vi "4_Analog_Meter_Reader(Evaluation).vi"() -> ()   [LabVIEW 2020]
uses:
  Controls/Regression_Report.ctl
  <vilib>/Ngene/DeepLTK/Toolkit/NN_Network/Controls/NN_Save_Before_Destroy_Options.ctl
  <vilib>/Ngene/DeepLTK/Toolkit/NN_Network/subVIs/NN_Predict/NN_Predict(In3D_Out1D).vi
  <vilib>/Ngene/DeepLTK/Toolkit/NN_Train/Eval_Loss/NN_Eval_Test_Error_Loss/NN_Eval(In3D_Out1D).vi
  <vilib>/Ngene/DeepLTK/Toolkit/Deep_Learning_Toolkit_by_Ngene.lvlib
panel:
  in  "Image Folder(Test)":path=path "D:/DeepLTK_Examples/Analog_Meter/Test/Images"
  in  "Labels (Test)":path=path "D:/DeepLTK_Examples/Analog_Meter/Test/Labels.csv"
  in  "NN Device":enum16{"CPU", "GPU"}(ring)=enum."GPU"
  in  "Image Folder(Train)":path=path "D:/DeepLTK_Examples/Analog_Meter/Train/Images"
  in  "Labels (Train)":path=path "D:/DeepLTK_Examples/Analog_Meter/Train/Labels.csv"
  out "Metrics (Test)":T1={"Graphs"=[{"Best Linear Fit"=[0.0, 0.7035179734230042, 1.407034993171692, 2.110553026199341, 2.814069986343384, 3.517587900161743, 4.221106052398682, 4.924623012542725, 5.628140926361084, 6.331657886505127, 7.035175800323486, 7.7386932373046875, 8.442211151123047, 9.145729064941406, 9.84924602508545, 10.552763938903809, 11.256280899047852, 11.959798812866211, 12.66331672668457, 13.366833686828613, 14.070351600646973, 14.773868560791016, 15.477387428283691, 16.180904388427734, 16.884422302246094, 17.587940216064453, 18.29145622253418, 18.99497413635254, 19.6984920501709, 20.402009963989258, 21.105527877807617, 21.809045791625977, 22.512563705444336, 23.216079711914062, 23.919597625732422, 24.62311553955078, 25.32663345336914, 26.0301513671875, 26.733667373657227, 27.437185287475586, 28.140703201293945, 28.844221115112305, 29.547739028930664, 30.251256942749023, 30.954774856567383, 31.65829086303711, 32.36180877685547, 33.06532669067383, 33.76884460449219, 34.47236251831055, 35.175880432128906, 35.879398345947266, 36.582916259765625, 37.28643035888672, 37.98994827270508, 38.69346618652344, 39.3969841003418, 40.100502014160156, 40.804019927978516, 41.507537841796875, 42.211055755615234, 42.914573669433594, 43.61809158325195, 44.32160949707031, 45.02512741088867, 45.728641510009766, 46.432159423828125, 47.135677337646484, 47.839195251464844, 48.5427131652832, 49.24623107910156, 49.94974899291992, 50.65326690673828, 51.35678482055664, 52.060302734375, 52.76382064819336, 53.46733856201172, 54.17085266113281, 54.87437057495117, 55.57788848876953, 56.28140640258789, 56.98492431640625, 57.68844223022461, 58.39196014404297, 59.09547805786133, 59.79899597167969, 60.50251388549805, 61.206031799316406, 61.909549713134766, 62.61306381225586, 63.31658172607422, 64.02010345458984, 64.72361755371094, 65.42713928222656, 66.13065338134766, 66.83416748046875, 67.53768920898438, 68.24120330810547, 68.9447250366211, 69.64823913574219, 70.35176086425781, 71.0552749633789, 71.75879669189453, 72.46231079101562, 73.16583251953125, 73.86934661865234, 74.57286071777344, 75.27638244628906, 75.97989654541016, 76.68341827392578, 77.38693237304688, 78.0904541015625, 78.7939682006836, 79.49748992919922, 80.20100402832031, 80.90452575683594, 81.60803985595703, 82.31156158447266, 83.01507568359375, 83.71858978271484, 84.42211151123047, 85.12562561035156, 85.82914733886719, 86.53266143798828, 87.2361831665039, 87.939697265625, 88.64321899414062, 89.34673309326172, 90.05024719238281, 90.75376892089844, 91.45728302001953, 92.16080474853516, 92.86431884765625, 93.56784057617188, 94.27135467529297, 94.9748764038086, 95.67839050292969, 96.38191223144531, 97.0854263305664, 97.78894805908203, 98.49246215820312, 99.19597625732422, 99.89949798583984, 100.60301208496094, 101.30653381347656, 102.01004791259766, 102.71356964111328, 103.41708374023438, 104.12060546875, 104.8241195678711, 105.52764129638672, 106.23115539550781, 106.9346694946289, 107.63819122314453, 108.34170532226562, 109.04522705078125, 109.74874114990234, 110.45226287841797, 111.15577697753906, 111.85929870605469, 112.56281280517578, 113.2663345336914, 113.9698486328125, 114.67337036132812, 115.37688446044922, 116.08039855957031, 116.78392028808594, 117.48743438720703, 118.19095611572266, 118.89447021484375, 119.59799194335938, 120.30150604248047, 121.0050277709961, 121.70854187011719, 122.41206359863281, 123.1155776977539, 123.819091796875, 124.52261352539062, 125.22612762451172, 125.92964935302734, 126.63316345214844, 127.33668518066406, 128.0402069091797, 128.74371337890625, 129.44723510742188, 130.1507568359375, 130.85427856445312, 131.5577850341797, 132.2613067626953, 132.96482849121094, 133.6683349609375, 134.37185668945312, 135.07537841796875, 135.77890014648438, 136.48240661621094, 137.18592834472656, 137.8894500732422, 138.5929718017578, 139.29647827148438, 140.0], "Array 3"=[3.275964, 3.249447, 2.547323, 2.4843557, 2.314022, 5.9284067, 5.9090176, 6.770803, 7.256697, 8.836181, 9.031486, 10.445968, 11.187589, 9.598534, 10.856343, 11.660367, 12.432229, 13.276137, 15.303519, 15.652077, 15.5077095, 15.784932, 16.294615, 17.2778, 18.094921, 18.929054, 19.75645, 20.359539, 20.938688, 22.076456, 22.729862, 23.16336, 23.454283, 24.118996, 25.31959, 26.342335, 26.424267, 26.912985, 27.571787, 28.408794, 29.294344, 30.003319, 30.542835, 31.343233, 32.022118, 32.687912, 33.300972, 34.221542, 34.977905, 35.367214, 36.47949, 37.113617, 37.63445, 37.84932, 38.15908, 40.29969, 40.538902, 40.899334, 41.505558, 42.122498, 42.90602, 43.561836, 44.778614, 44.878468, 45.97382, 46.838966, 47.30163, 47.776108, 48.446632, 48.980473, 49.125286, 50.393486, 51.820633, 52.201366, 52.935173, 53.599346, 53.993423, 54.49489, 55.118916, 56.33319, 57.0652, 57.44734, 58.025818, 58.567043, 59.989807, 60.53097, 61.444412, 61.949356, 62.503365, 63.341396, 63.55453, 64.01239, 64.65186, 65.49459, 66.332726, 67.896835, 68.46354, 69.26983, 69.97261, 70.04088, 70.97165, 71.28301, 71.93522, 72.59067, 73.28446, 74.66231, 75.173546, 76.099106, 76.66713, 77.37499, 77.719444, 78.54047, 79.172646, 79.37848, 80.14726, 80.78076, 82.376884, 82.99884, 83.60962, 84.0593, 84.44566, 85.8675, 86.52428, 87.15648, 87.46964, 88.227005, 88.80414, 89.10876, 90.562164, 91.68537, 92.0146, 92.772575, 93.30528, 93.95562, 94.22434, 95.10878, 96.05684, 96.24298, 97.40361, 97.8748, 98.68413, 99.06965, 99.799774, 100.4482, 100.78638, 103.01562, 103.53611, 103.72109, 103.98403, 104.65476, 105.434685, 106.22847, 106.88888, 107.90816, 108.23753, 108.73593, 109.4663, 110.35882, 111.21342, 112.03596, 113.082985, 113.7248, 114.333855, 114.45049, 114.43153, 115.7888, 117.253975, 117.98268, 118.36474, 118.62209, 118.934456, 120.12705, 121.109024, 121.56967, 122.25218, 123.0601, 123.699196, 124.492615, 124.93293, 125.44291, 125.92214, 126.38807, 128.61964, 128.89961, 129.13136, 130.06342, 131.20547, 129.63286, 130.81374, 132.5757, 133.68027, 133.92395, 134.80855, 135.73024, 136.06657, 139.30591, 139.29033, 138.47128, 138.88876, 137.8662]}, {"Best Linear Fit"=[1.766071485527795, 1.7391815000363957, 1.027179073734446, 0.9633258753149123, 0.7905957977694533, 4.455831861176305, 4.436169919258462, 5.310079941353025, 5.802810275390483, 7.404515815247787, 7.602568464366818, 9.03695117830171, 9.789006192056242, 8.177594436072901, 9.453100419690095, 10.268436113561304, 11.051157606004281, 11.906939010115426, 13.962844498937155, 14.316305887438006, 14.169907541684072, 14.451030468945696, 14.967883939041325, 15.964901353263414, 16.793519084924192, 17.63938779882541, 18.478424976761474, 19.089998311952737, 19.67729571059284, 20.831070957157024, 21.49366998609032, 21.933267333510877, 22.228282533442304, 22.902347401900364, 24.119832717308366, 25.15696703058294, 25.24005181510145, 25.73564570774491, 26.403716541674086, 27.25250007004289, 28.150508567356564, 28.869458097085143, 29.41656509770145, 30.228223908823576, 30.916659760356698, 31.59182131083408, 32.2135065571312, 33.14702859687304, 33.91403291455586, 34.30881909967721, 35.43674205017392, 36.079792286921524, 36.60795202640683, 36.82584552941335, 37.13996465933568, 39.31069101481531, 39.55326856708212, 39.91877121468577, 40.533524347478036, 41.15914372292382, 41.953690813014305, 42.618732715652015, 43.85262957768074, 43.95388794994801, 45.06465082482669, 45.94196936171588, 46.41114037417247, 46.89229558731992, 47.572253912767174, 48.11360478341963, 48.26045572810217, 49.54649817609371, 50.99372386817375, 51.37981396447875, 52.12394462861571, 52.79746212315584, 53.19708376691617, 53.70560380759337, 54.33841060876015, 55.56976982209513, 56.312078485416926, 56.69959214074524, 57.28621064099242, 57.835050669984945, 59.27783160848402, 59.826609743605964, 60.752901805590795, 61.264949796891, 61.82675272340291, 62.676574908287364, 62.8927083043493, 63.3570090428647, 64.00547886165488, 64.86006300620701, 65.70998963699807, 67.29610517465741, 67.87078202624977, 68.68841553006622, 69.4010847661145, 69.47031306035711, 70.41417911321948, 70.72992295724451, 71.39130538478425, 72.05597592419848, 72.75953128780398, 74.15676220592383, 74.67519300262748, 75.61377486628916, 76.18979017283279, 76.90761207360676, 77.25691013221943, 78.0894832690469, 78.73055677030288, 78.9392861120968, 79.71888583244245, 80.36129778864971, 81.97987666142775, 82.61058293936175, 83.22995490224598, 83.6859657304707, 84.0777616679697, 85.51960259330936, 86.18561932440869, 86.82671603586616, 87.14428574907326, 87.91230357888682, 88.49755654561436, 88.8064611169404, 90.28031664683706, 91.41932633690124, 91.75318961153828, 92.52182638005762, 93.06202834573746, 93.7215152734907, 93.99401851218246, 94.89089938054153, 95.8522968722454, 96.04105770404375, 97.21801607350669, 97.6958367543767, 98.51654947825446, 98.907494375033, 99.64789206510066, 100.30543707266449, 100.64837553607518, 102.90897952836937, 103.43679498319958, 103.62437983145693, 103.89101862591134, 104.57118584317179, 105.36208119489811, 106.1670341919797, 106.83673360837848, 107.87035351031423, 108.2043637828939, 108.70977365657451, 109.45041892212448, 110.35549299160145, 111.22211549398119, 112.05622824083932, 113.11798664368706, 113.7688316397607, 114.38645510080107, 114.50473428747758, 114.48550850392897, 115.86187345092985, 117.34765902438062, 118.08661768195732, 118.4740501015805, 118.73502560687692, 119.05178296303268, 120.26115824721138, 121.25694552075572, 121.7240740354832, 122.4161867697654, 123.23546819788604, 123.88355891671891, 124.68814055057702, 125.13465066966786, 125.65180490529085, 126.13778010360964, 126.6102624381422, 128.87323387098604, 129.15714105533198, 129.39215208192053, 130.33731790606504, 131.4954450654043, 129.900703069533, 131.09819473056052, 132.88494698643558, 134.0050558357717, 134.25216711405844, 135.14921045382775, 136.0838697934415, 136.42493596726717, 139.70984483397496, 139.69404642350966, 138.8634771007422, 139.28683117550267, 138.24987674128948], "Array 3"=[3.275964, 3.249447, 2.547323, 2.4843557, 2.314022, 5.9284067, 5.9090176, 6.770803, 7.256697, 8.836181, 9.031486, 10.445968, 11.187589, 9.598534, 10.856343, 11.660367, 12.432229, 13.276137, 15.303519, 15.652077, 15.5077095, 15.784932, 16.294615, 17.2778, 18.094921, 18.929054, 19.75645, 20.359539, 20.938688, 22.076456, 22.729862, 23.16336, 23.454283, 24.118996, 25.31959, 26.342335, 26.424267, 26.912985, 27.571787, 28.408794, 29.294344, 30.003319, 30.542835, 31.343233, 32.022118, 32.687912, 33.300972, 34.221542, 34.977905, 35.367214, 36.47949, 37.113617, 37.63445, 37.84932, 38.15908, 40.29969, 40.538902, 40.899334, 41.505558, 42.122498, 42.90602, 43.561836, 44.778614, 44.878468, 45.97382, 46.838966, 47.30163, 47.776108, 48.446632, 48.980473, 49.125286, 50.393486, 51.820633, 52.201366, 52.935173, 53.599346, 53.993423, 54.49489, 55.118916, 56.33319, 57.0652, 57.44734, 58.025818, 58.567043, 59.989807, 60.53097, 61.444412, 61.949356, 62.503365, 63.341396, 63.55453, 64.01239, 64.65186, 65.49459, 66.332726, 67.896835, 68.46354, 69.26983, 69.97261, 70.04088, 70.97165, 71.28301, 71.93522, 72.59067, 73.28446, 74.66231, 75.173546, 76.099106, 76.66713, 77.37499, 77.719444, 78.54047, 79.172646, 79.37848, 80.14726, 80.78076, 82.376884, 82.99884, 83.60962, 84.0593, 84.44566, 85.8675, 86.52428, 87.15648, 87.46964, 88.227005, 88.80414, 89.10876, 90.562164, 91.68537, 92.0146, 92.772575, 93.30528, 93.95562, 94.22434, 95.10878, 96.05684, 96.24298, 97.40361, 97.8748, 98.68413, 99.06965, 99.799774, 100.4482, 100.78638, 103.01562, 103.53611, 103.72109, 103.98403, 104.65476, 105.434685, 106.22847, 106.88888, 107.90816, 108.23753, 108.73593, 109.4663, 110.35882, 111.21342, 112.03596, 113.082985, 113.7248, 114.333855, 114.45049, 114.43153, 115.7888, 117.253975, 117.98268, 118.36474, 118.62209, 118.934456, 120.12705, 121.109024, 121.56967, 122.25218, 123.0601, 123.699196, 124.492615, 124.93293, 125.44291, 125.92214, 126.38807, 128.61964, 128.89961, 129.13136, 130.06342, 131.20547, 129.63286, 130.81374, 132.5757, 133.68027, 133.92395, 134.80855, 135.73024, 136.06657, 139.30591, 139.29033, 138.47128, 138.88876, 137.8662]}, {"Best Linear Fit"=[0.0, 140.0], "Array 3"=[0.0, 140.0]}], "y=k*x+b"="y = 0.986*x + 1.534", "R"=0.99991375, "R^2"=0.9998275, "MAE"=0.73401445, "MSE"=0.9198636} {"R" format="%#_7g"}
  out "Metrics (Train)":T1={"Graphs"=[{"Best Linear Fit"=array[1000 elements], "Array 3"=array[1000 elements]}, {"Best Linear Fit"=array[1000 elements], "Array 3"=array[1000 elements]}, {"Best Linear Fit"=[0.0, 140.0], "Array 3"=[0.0, 140.0]}], "y=k*x+b"="y = 0.987*x + 1.447", "R"=0.9999118, "R^2"=0.9998236, "MAE"=0.71916497, "MSE"=0.8626691} {"R" format="%#_7g"}
  in  "Network Configuration File Path":path
  in  "Weight File Path":path
  # "Performs evaluation of a trained model over Training and Tests Datasets\nInstructions:\n1. Provide paths to Train and Test datasets \n2. Provide model files (.cfg and .bin).\n2. Run the VI\n3. Drag and drop image on \"Input Image\"\n4. Observe rge prediction result."
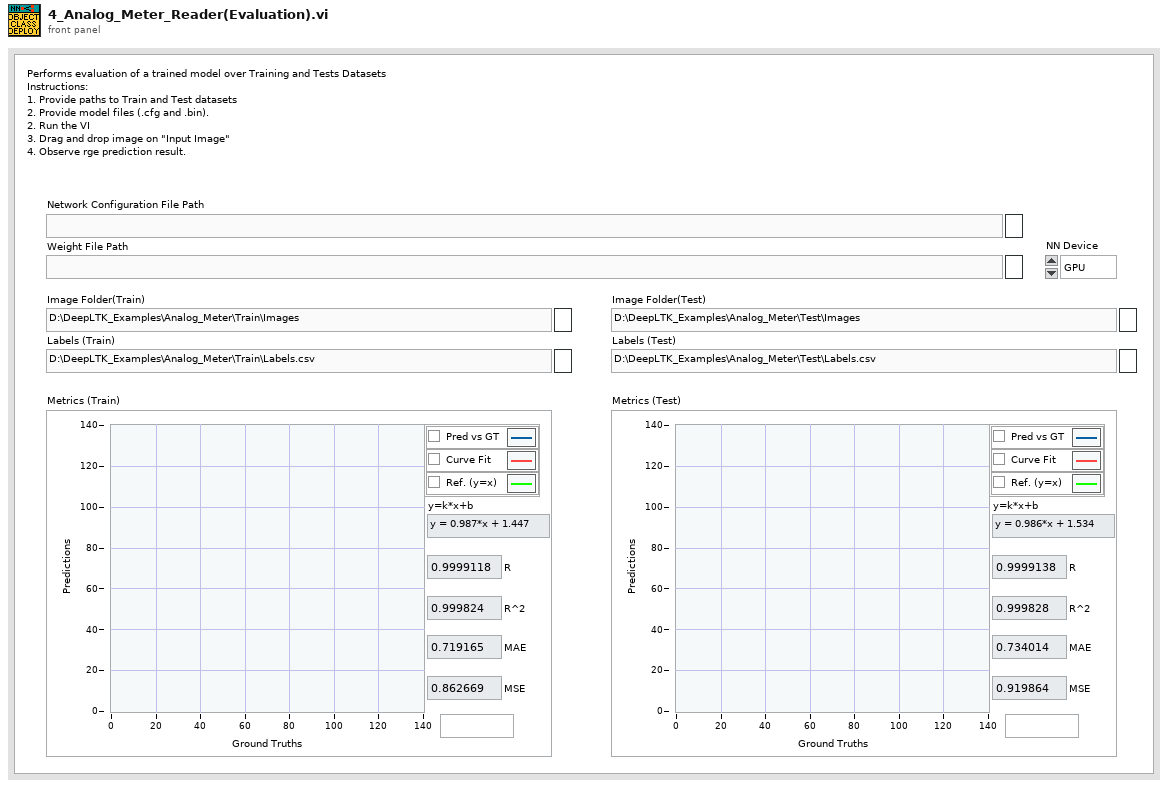
[diagram p1: front panel]
types:
  T1 = typedef "Regression_Report.ctl" = cluster{"Graphs":cluster{"Best Linear Fit":dbl[], "Array 3":sgl[]}[], "y=k*x+b":string, "R":sgl, "R^2":sgl, "MAE":sgl, "MSE":sgl}
  T2 = typedef "Deep_Learning_Toolkit_by_Ngene.lvlib/NN_Save_Before_Destroy_Options.ctl" = cluster{"CFG?":bool, "Weights?":bool, "Render?":bool}
  T3 = typedef "Deep_Learning_Toolkit_by_Ngene.lvlib/NN_Config_Params.ctl" = cluster{"Name":string, "mBatch":i32, "NN_Train_Params":T4, "LR_Decay_Policy":T7, "Labels":string[], "Loss":T9}
  T4 = typedef "Deep_Learning_Toolkit_by_Ngene.lvlib/NN_Train_Params.ctl" = cluster{"Optimizer":T5, "Beta_1":sgl, "Beta_2":sgl, "Weight Decay(L1)":sgl, "Weight Decay(L2)":sgl, "Data_Sampling":T6}
  T5 = typedef "Deep_Learning_Toolkit_by_Ngene.lvlib/NN_Train_Optimizer.ctl" = enum16{"SGD", "Adam", "Adagrad", "Adadelta", "RMSProp", "Nesterov"}
  T6 = typedef "Deep_Learning_Toolkit_by_Ngene.lvlib/NN_Train_Data_Sampling.ctl" = enum16{"Random", "Sequential"}
  T7 = typedef "Deep_Learning_Toolkit_by_Ngene.lvlib/NN_LR_Policy_Cfg.ctl" = cluster{"Policy_Type":T8, "LR0":dbl, "k":sgl, "WarmUp_Policy":enum16{"Step", "Ramp"}, "WarmUp_Iter":i32, "WarmUp_Ratio":sgl}
  T8 = typedef "Deep_Learning_Toolkit_by_Ngene.lvlib/NN_LR_Policy_Type.ctl" = enum16{"Manual", "Step", "Exp", "1/t"}
  T9 = typedef "Deep_Learning_Toolkit_by_Ngene.lvlib/NN_Loss_Config_Params.ctl" = cluster{"Loss_Type":T10, "Loss_Conf_Params":variant}
  T10 = typedef "Deep_Learning_Toolkit_by_Ngene.lvlib/NN_Loss_Type.ctl" = enum16{"None", "MSE", "CrossEntropy", "YOLO_v2"}
  T11 = typedef "Deep_Learning_Toolkit_by_Ngene.lvlib/NN_Layer_Config_Params.ctl" = cluster{"Layer_Type":T12, "Layer_Conf_Params":variant}
  T12 = typedef "Deep_Learning_Toolkit_by_Ngene.lvlib/NN_Layer_Type.ctl" = enum16{"Input1D", "Input3D", "Conv2D", "Conv2D_Adv", "MaxPool", "AvgPool", "UpSample", "DropOut3D", "ShortCut", "Concat", "SoftMax3D", "FC", "DropOut", "Softmax", "Flatten", "YOLO_v2", "Unsupported"}
  T13 = typedef "Deep_Learning_Toolkit_by_Ngene.lvlib/NN.ctl" = cluster{"Name":string, "No of Layers":i32, "mBatch":i32, "Layers":T14[], "Dimty":T15, "Dims_In":T16, "Dims_Out":T16, "Working_Dir":path, "Train?":bool, "Train_Params":T4, "LR_Update_Policy":T7, "Session Data":T17, "Ground_truth":T18, "NNg_hdls":T20, "NN_Device":T21, "GPU Id":i32, "Labels":string[], "Receptive Field":T22[], "Loss_Type":T10, "Loss_Cfg_Prms":variant}
  T14 = typedef "Deep_Learning_Toolkit_by_Ngene.lvlib/NN_Layer_ref.ctl" = refnum<data-value>
  T15 = typedef "Deep_Learning_Toolkit_by_Ngene.lvlib/NN_In_Out_Dim-ty.ctl" = enum8{"In1D_Out1D", "In3D_Out1D", "In3D_Out3D", "In3D_OutBBox"}
  T16 = typedef "Deep_Learning_Toolkit_by_Ngene.lvlib/NN_Dims(C,H,W).ctl" = cluster{"C":i32, "H":i32, "W":i32}
  T17 = typedef "Deep_Learning_Toolkit_by_Ngene.lvlib/NN_Train_Session_Data.ctl" = cluster{"Epochs":sgl, "Tot_Iter":i32, "LR":sgl, "LR_iter":i32}
  T18 = typedef "Deep_Learning_Toolkit_by_Ngene.lvlib/NN_Ground_truth.ctl" = cluster{"Y":variant, "Y_idx":T19}
  T19 = typedef "Deep_Learning_Toolkit_by_Ngene.lvlib/NN_Data_ref(1D_I32).ctl" = refnum<data-value>
  T20 = typedef "Deep_Learning_Toolkit_by_Ngene.lvlib/nng_cuda_handles.ctl" = cluster{"cudnn":u64, "cublas":u64, "stream":u64, "curand":u64}
  T21 = typedef "Deep_Learning_Toolkit_by_Ngene.lvlib/NN_Device.ctl" = enum16{"CPU", "GPU"}
  T22 = typedef "Deep_Learning_Toolkit_by_Ngene.lvlib/NN_Dims(V,H).ctl" = cluster{"V":i32, "H":i32}
  T23 = typedef "Deep_Learning_Toolkit_by_Ngene.lvlib/NN_DataSets_All(In3D_Out1D).ctl" = cluster{"Train":T24, "Validation":T24, "Test":T24}
  T24 = typedef "Deep_Learning_Toolkit_by_Ngene.lvlib/NN_DataSet(In3D_Out1D).ctl" = cluster{"Inputs Ref.":T25, "Outputs Ref.":T26, "Dataset_Size":i32, "Outputs_idx Ref.":T19, "Dims_In":T16, "Dims_Out":i32, "Labels":string[], "File Paths":path[]}
  T25 = typedef "Deep_Learning_Toolkit_by_Ngene.lvlib/NN_Data_ref(4D_SGL).ctl" = refnum<data-value>
  T26 = typedef "Deep_Learning_Toolkit_by_Ngene.lvlib/NN_Data_ref(2D_SGL).ctl" = refnum<data-value>
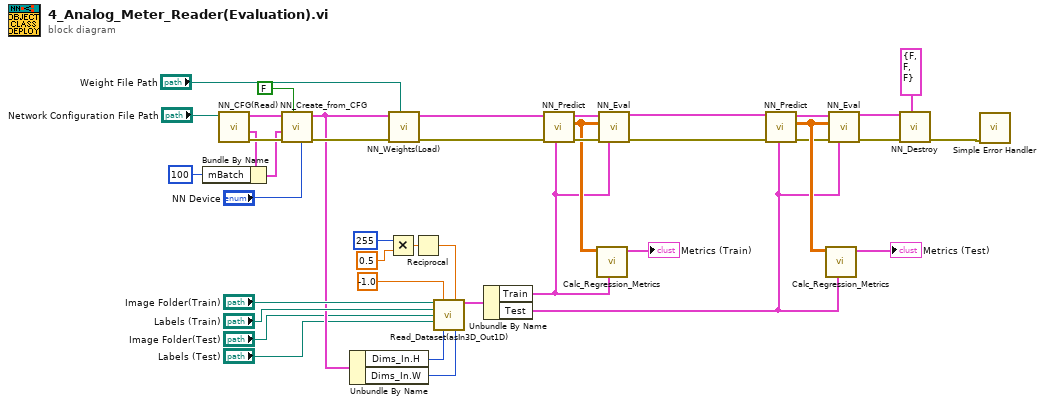
[diagram p0: block diagram]
diagram:
  n1 = call <vilib>:"NN_CFG(Read).vi"("CFG file path"="Network Configuration File Path") -> ("error out"=w41:errorcluster, "Net_Cfg"=w35:T3, "Layer_Cfg"=w34:T11[])  [unwired: 8 in]
  n2 = Bundle By Name(cluster=w35, "mBatch"=100) -> (w32:T3)
  n3 = call <vilib>:"NN_Create_from_CFG.vi"("NN_Device"="NN Device", "Train? (false)"=FALSE, "error in (no error)"=w41, "Net_Cfg"=w32, "Layer_Cfg"=w34) -> ("error out"=w37:errorcluster, "NN out"=w9:T13)  [unwired: 5 in]
  n4 = Unbundle By Name(w9) -> ("Dims_In.H"=w8:i32, "Dims_In.W"=w7:i32)
  n5 = Multiply(x=u16 255 ("Shift"), y=sgl 0.5 ("Scale")) -> (x*y=w27:sgl)
  n6 = call <vilib>:"NN_Weights(Load).vi"("Weight File Path"="Weight File Path", "error in (no error)"=w37, "NN in"=w9) -> ("error out"=w21:errorcluster, "NN out"=w33:T13)  [unwired: 7 in]
  n7 = Reciprocal(x=w27) -> (1/x=w26:sgl)
  n8 = call "Read_Dataset(asIn3D_Out1D).vi"("Image Folder Path(Train)"="Image Folder(Train)", "Norm. Shift"=sgl -1.0 ("Scale"), "Norm. Scale"=w26, "Label File Path(Train)"="Labels (Train)", "Image Folder Path(Test)"="Image Folder(Test)", "Label File Path(Test)"="Labels (Test)", "Img Heigth"=w8, "Img Width"=w7) -> ("Datasets"=w22:T23)  [unwired: 6 in, 1 out]
  n9 = Unbundle By Name(w22) -> ("Train"=w6:T24, "Test"=w5:T24)
  n10 = call-poly <vilib>:"NN_Predict.vi"("Dataset"=w6, "error in (no error)"=w21, "NN in"=w33) -> ("error out"=w24:errorcluster, "Predictions"=w23:sgl[][], "NN out"=w25:T13)  [unwired: 6 in]
  n11 = call "Calc_Regression_Metrics.vi"("Dataset"=w6, "Predictions"=w23) -> ("Metrics"=→"Metrics (Train)":T1)  [unwired: 9 in]
  n12 = call-poly <vilib>:"NN_Eval.vi"("NN in"=w25, "Predictions"=w23, "error in (no error)"=w24, "Dataset"=w6) -> ("NN out"=w17:T13, "error out"=w16:errorcluster)  [unwired: 7 in, 3 out]
  n13 = call-poly <vilib>:"NN_Predict.vi"("Dataset"=w5, "error in (no error)"=w16, "NN in"=w17) -> ("error out"=w19:errorcluster, "Predictions"=w20:sgl[][], "NN out"=w18:T13)  [unwired: 6 in]
  n14 = call "Calc_Regression_Metrics.vi"("Dataset"=w5, "Predictions"=w20) -> ("Metrics"=→"Metrics (Test)":T1)  [unwired: 9 in]
  n15 = call-poly <vilib>:"NN_Eval.vi"("NN in"=w18, "Predictions"=w20, "error in (no error)"=w19, "Dataset"=w5) -> ("NN out"=w15:T13, "error out"=w14:errorcluster)  [unwired: 7 in, 3 out]
  n16 = call <vilib>:"NN_Destroy.vi"("Save (T, T, T)"=T2 {"CFG?"=FALSE, "Weights?"=FALSE, "Render?"=FALSE} ("Save_Config"), "error in (no error)"=w14, "NN in"=w15) -> ("error out"=w39:errorcluster)  [unwired: 8 in]
  n17 = call <vilib>:"Simple Error Handler.vi"("error in (no error)"=w39) -> ()  [unwired: 4 in, 5 out]
